vi "FindEdgePoints.vi"(0 "X1":i32, 1 "Image in":T1, 2 "Y1":i32, 3 "X2":i32, 4 "error in (no error)":errorcluster, 5 "Y2":i32) -> (6 "Image out":T1, 7 "Edge point":T2[](array[typedef]) {"Distance (Real-World)" format="%.2f"; "Location (Real-World)"."Y" format="%.2g"; "Location (Real-World)"."X" format="%.2f"; "Noise" format="%.2f"; "Location (Pixel)"."Y" format="%.2g"; "Location (Pixel)"."X" format="%.2f"; "Strength" format="%.2f"; "Distance (Pixel)" format="%.2f"}, 8 "error out":errorcluster)   [LabVIEW 2014]
uses:
  <vilib>/vision/NI_Vision_Development_Module.lvlib
  <vilib>/vision/Measure.llb/Edge Polarity.ctl
  <vilib>/vision/Measure.llb/Edge Options.ctl
  <vilib>/vision/Measure.llb/Edge New.ctl
  <vilib>/vision/Image Controls.llb/IMAQ Image.ctl
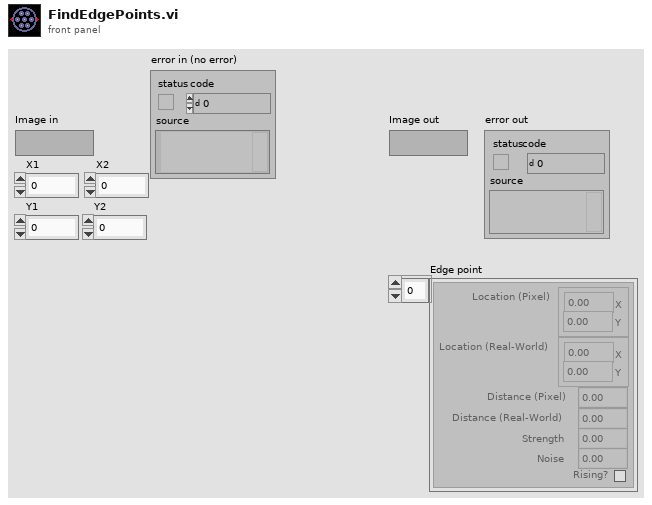
[diagram p1: front panel]
types:
  T1 = typedef "IMAQ Image.ctl" = refnum<image>
  T2 = typedef "Edge New.ctl" = cluster{"Location (Pixel)":cluster{"X":sgl, "Y":sgl}, "Location (Real-World)":cluster{"X":sgl, "Y":sgl}, "Distance (Pixel)":dbl, "Distance (Real-World)":dbl, "Strength":dbl, "Noise":dbl, "Rising?":bool}
  T3 = typedef "Edge Options.ctl" = cluster{"Edge Polarity":T4, "Kernel Size":u32, "Width":u32, "Minimum Edge Strength":sgl, "Interpolation Type":enum32{"Zero Order", "Bilinear", "Quadratic", "Cubic", "Bilinear Fixed"}, "Data Processing Method":enum32{"Average", "Median"}}
  T4 = typedef "Edge Polarity.ctl" = u32
  T5 = enum16{"Get First Edge", "Get First + Last Edge", "Get All Edges", "Get Best Edge"}
  T6 = typedef "ROI Descriptor" = cluster{"Global Rectangle":i32[], "Contours":cluster{"ID":enum32{"External", "Internal"}, "Type":u32, "Coordinates":i32[]}[]}
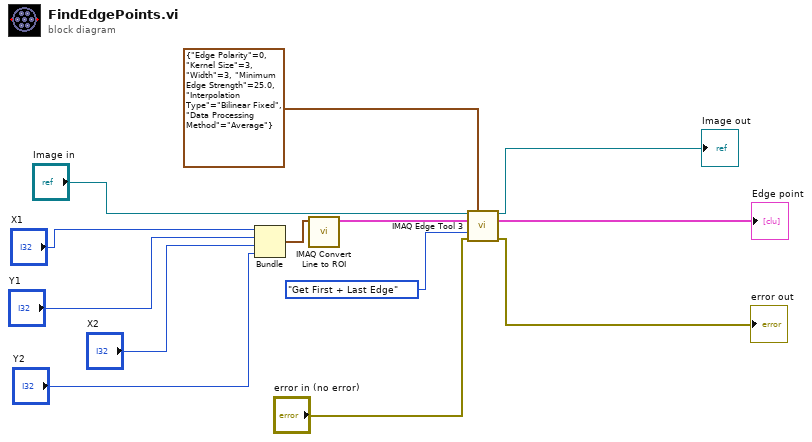
[diagram p0: block diagram]
diagram:
  n1 = Bundle("X1"="X1", "Y1"="Y1", "X2"="X2", "Y2"="Y2") -> (w7:cluster{"X1":i32, "Y1":i32, "X2":i32, "Y2":i32})  [unwired: 1 in]
  n2 = call "IMAQ Convert Line to ROI"("Line"=w7) -> ("ROI Descriptor"=w9:T6)  [unwired: 8 in, 1 out]
  n3 = call "IMAQ Edge Tool 3"("Image"="Image in", "Edge Options"=T3 {"Edge Polarity"=0, "Kernel Size"=3, "Width"=3, "Minimum Edge Strength"=25.0, "Interpolation Type"=enum."Bilinear Fixed", "Data Processing Method"=enum."Average"}, "ROI Descriptor"=w9, "Process"=T5."Get First + Last Edge", "error in (no error)"="error in (no error)") -> ("Image (duplicate)"=→"Image out":T1, "Edge Information"=→"Edge point":T2[], "error out"=→"error out":errorcluster)  [unwired: 6 in, 2 out]
